vi "PadRect.vi"(9 "Padding":i16, 10 "Rectagle":T1) -> (2 "Padded Rectangle":T1)   [LabVIEW 2013, in "BarCodes.lvlib"]
doc: "Adds or subtracts the appropriate padding to a rectangle. A positive padding makes a smaller rectangle. A negative padding makes a larger rectangle."
uses:
  BarCodes.lvlib
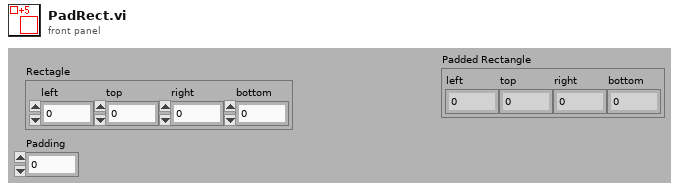
[diagram p1: front panel]
types:
  T1 = cluster{"left":i16, "top":i16, "right":i16, "bottom":i16}
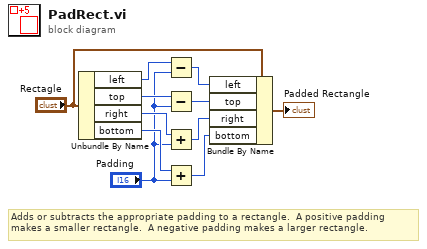
[diagram p0: block diagram]
diagram:
  # "Adds or subtracts the appropriate padding to a rectangle.  A positive padding\nmakes a smaller rectangle.  A negative padding makes a larger rectangle."
  n1 = Unbundle By Name("Rectagle") -> ("left"=w11:i16, "top"=w10:i16, "right"=w9:i16, "bottom"=w8:i16)
  n2 = Subtract(x=w11, y="Padding") -> (x-y=w5:i16)
  n3 = Subtract(x=w10, y="Padding") -> (x-y=w4:i16)
  n4 = Add(x=w9, y="Padding") -> (x+y=w3:i16)
  n5 = Add(x=w8, y="Padding") -> (x+y=w2:i16)
  n6 = Bundle By Name(cluster="Rectagle", "left"=w5, "top"=w4, "right"=w3, "bottom"=w2) -> (→"Padded Rectangle":T1)
